vi "pythonHyperstack_CAllocated.vi"(1 "refresh_time":dbl=0.1, 2 "shape":i32[](array[numeric]), 3 "ptr":i64) -> (0 "ptr out":i64)   [LabVIEW 2017]
uses:
  globalUtilities.vi
  dll/wormUtilities/x64/Release/wormUtilities.dll
panel:
  out "return type":dbl
  out "Array 2":dbl[](array[numeric])
  out "Array":dbl[](array[numeric])
  out "result":bool
  out "shape 2":i32[](array[numeric])
  out "out":sgl[](array[numeric])
  out "Numeric":i32
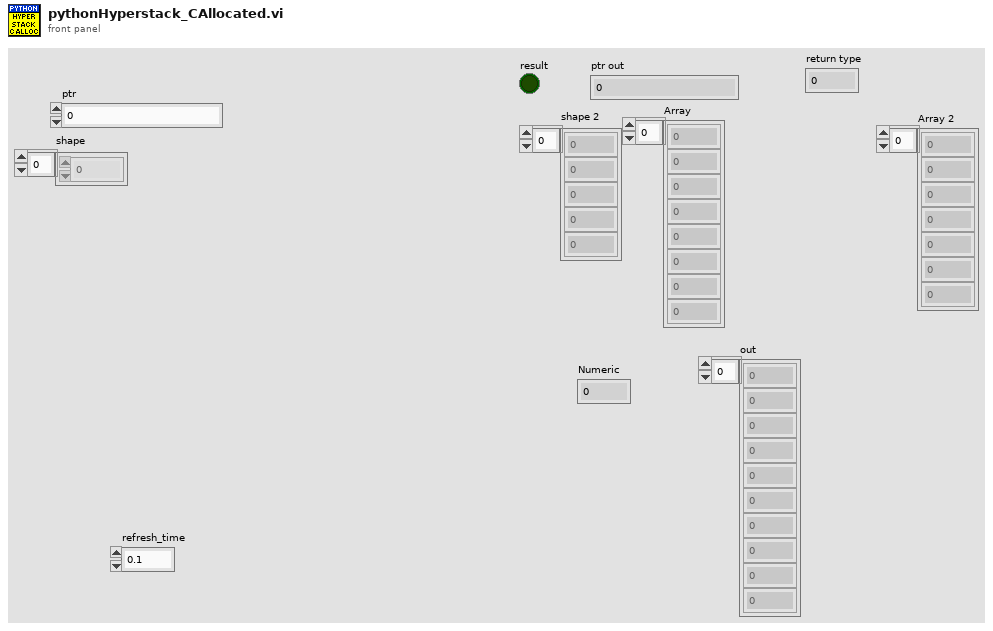
[diagram p1: front panel]
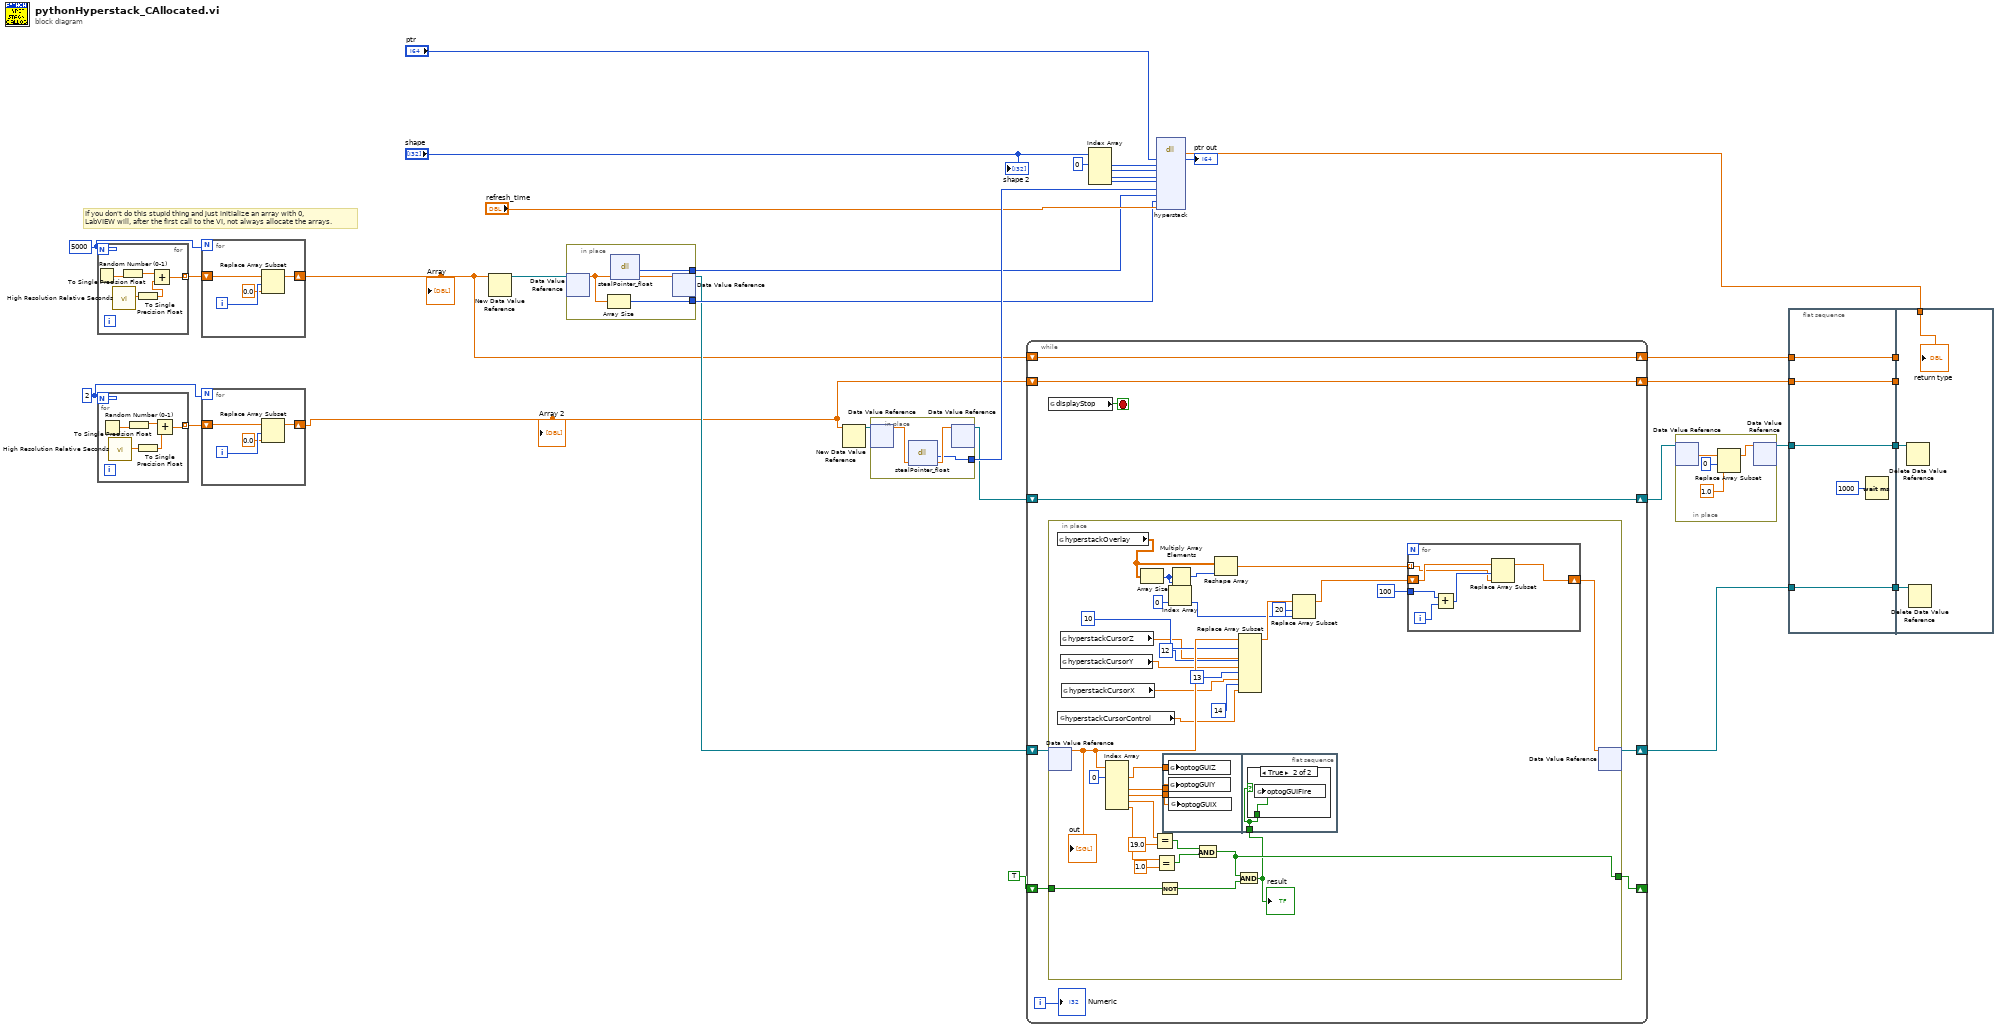
[diagram p0: block diagram]
diagram:
  w18 = 2
  w17 = 5000
  # "If you don't do this stupid thing and just initialize an array with 0, \nLabVIEW will, after the first call to the VI, not always allocate the arrays."
  n1 = for {
    N: w17 -> [_]
    tunnel: [w36] -> w22 mode=indexing
    n2 = Random Number (0-1)() -> (number: 0 to 1=w38:dbl)
    n3 = call <vilib>:"High Resolution Relative Seconds.vi"() -> ("relative seconds"=w35:dbl)
    n4 = To Single Precision Float(number=w38) -> (single precision float=w37:sgl)
    n5 = To Single Precision Float(number=w35) -> (single precision float=w34:sgl)
    n6 = Add(x=w37, y=w34) -> (x+y=w36:sgl)
  }
  n7 = for {
    N: w18 -> [_]
    tunnel: [w41] -> w20 mode=indexing
    n8 = Random Number (0-1)() -> (number: 0 to 1=w43:dbl)
    n9 = call <vilib>:"High Resolution Relative Seconds.vi"() -> ("relative seconds"=w40:dbl)
    n10 = To Single Precision Float(number=w43) -> (single precision float=w42:sgl)
    n11 = To Single Precision Float(number=w40) -> (single precision float=w39:sgl)
    n12 = Add(x=w42, y=w39) -> (x+y=w41:sgl)
  }
  n13 = for {
    N: w17 -> [_]
    shift-right: [w44] -> w21
    shift-left: w22 -> [w47]
    i -> [w46]
    n14 = Replace Array Subset(array=w47, new element=sgl 0.0 ("new element/subarray"), index=w46) -> (w44:sgl[])
  }
  "Array" <- w21
  n15 = for {
    N: w18 -> [_]
    shift-right: [w48] -> w19
    shift-left: w20 -> [w51]
    i -> [w50]
    n16 = Replace Array Subset(array=w51, new element=sgl 0.0 ("new element/subarray"), index=w50) -> (w48:sgl[])
  }
  "Array 2" <- w19
  n17 = New Data Value Reference(data value=w21) -> (data value reference=w26:refnum<data-value>)  [unwired: 1 in, 1 out]
  n18 = in-place {
    in-place-border: [w54] -> w28
    in-place-border: [w52] -> w27
    n19 = in-place-dvr #1(w26) -> (w53:sgl[])  [unwired: 1 out]
    n20 = Array Size(array=w53) -> (size(s)=w52:i32)
    n21 = dll-call lib="C:/Users/francesco/dev/pump-probe/dll/wormUtilities/x64/Release/wormUtilities.dll" fn="stealPointer_float"("A"=w53) -> ("return type"=w54:i64, "A"=w55:sgl[])  [unwired: 3 in, 2 out]
    n22 = in-place-dvr #1(w55) -> (w24:refnum<data-value>)  [unwired: 1 out]
  }
  n23 = New Data Value Reference(data value=w19) -> (data value reference=w32:refnum<data-value>)  [unwired: 1 in, 1 out]
  n24 = in-place {
    in-place-border: [w56] -> w33
    n25 = in-place-dvr #2(w32) -> (w57:sgl[])  [unwired: 1 out]
    n26 = dll-call lib="C:/Users/francesco/dev/pump-probe/dll/wormUtilities/x64/Release/wormUtilities.dll" fn="stealPointer_float"("A"=w57) -> ("return type"=w56:i64, "A"=w58:sgl[])  [unwired: 3 in, 2 out]
    n27 = in-place-dvr #2(w58) -> (w31:refnum<data-value>)  [unwired: 1 out]
  }
  n28 = while {
    shift-right: [w63] -> w25
    shift-left: w24 -> [w65]
    shift-right: [w66] -> w30
    shift-left: w31 -> [w66]
    shift-right: [w62] -> w15
    shift-left: w21 -> [w62]
    shift-right: [w61] -> w14
    shift-left: w19 -> [w61]
    shift-right: [w60] -> _
    shift-left: TRUE -> [w59]
    i -> [w64]
    stop <- w67 stop-if-true
    n29 = global read "globalUtilities.vi" "displayStop"() -> (w67:bool)
    n30 = in-place {
      in-place-border: [w89] -> w60
      in-place-border: w59 -> [w91]
      n31 = in-place-dvr #3(w65) -> (w87:sgl[])  [unwired: 1 out]
      "out" <- w87
      n32 = global read "globalUtilities.vi" "hyperstackOverlay"() -> (w77:dbl[][])
      n33 = global read "globalUtilities.vi" "hyperstackCursorControl"() -> (w79:sgl)
      n34 = global read "globalUtilities.vi" "hyperstackCursorY"() -> (w81:sgl)
      n35 = global read "globalUtilities.vi" "hyperstackCursorZ"() -> (w82:sgl)
      n36 = global read "globalUtilities.vi" "hyperstackCursorX"() -> (w80:sgl)
      n37 = Index Array(array=w87, index #1=0 ("index")) -> (element #1=w100:sgl, element #3=w99:sgl, element #4=w98:sgl, element #5=w97:sgl, element #6=w95:sgl)  [unwired: 5 in, 1 out]
      n38 = Array Size(array=w77) -> (size(s)=w73:i32[])
      n39 = Equal?(x=w97, y=sgl 19.0) -> (x = y?=w93:bool)
      n40 = Equal?(x=w95, y=sgl 1.0) -> (x = y?=w92:bool)
      n41 = Not(x=w91) -> (.not. x?=w90:bool)
      n42 = flat-sequence {
        tunnel: w100 -> [w110]
        tunnel: w99 -> [w109]
        tunnel: w98 -> [w108]
        tunnel: w88 -> [w111]
        frame #0 {
          n43 = global write "globalUtilities.vi" "optogGUIZ"(w110) -> ()
          n44 = global write "globalUtilities.vi" "optogGUIY"(w109) -> ()
          n45 = global write "globalUtilities.vi" "optogGUIX"(w108) -> ()
        }
        frame #1 {
          n46 = case shown="True" w111 {
            tunnel: w111 -> [_ w112]
            frame False {
            }
            frame True {
              n47 = global write "globalUtilities.vi" "optogGUIFire"(w112) -> ()
            }
          }
        }
      }
      n48 = Index Array(array=w73, index=0) -> (element=w70:i32)
      n49 = Multiply Array Elements(1:w73) -> (0:w78:i32)
      n50 = Compound Arithmetic op=AND(w93, w92) -> (w89:bool)
      n51 = Reshape Array(w77, w78) -> (w76:dbl[])
      n52 = And(x=w89, y=w90) -> (x .and. y?=w88:bool)
      "result" <- w88
      n53 = Replace Array Subset(array=w87, new element #1=w82, index #1=10 ("index"), new element #2=w81, index #2=12 ("index"), new element #3=w80, index #3=13 ("index"), new element #4=w79, index #4=14 ("index")) -> (w71:sgl[])
      n54 = Replace Array Subset(array=w71, new element=w70, index=20) -> (w68:sgl[])
      n55 = for {
        tunnel: w76 -> [w103] mode=indexing
        tunnel: 100 -> [w106]
        shift-right: [w102] -> w74
        shift-left: w68 -> [w105]
        i -> [w107]
        n56 = Add(x=w106, y=w107) -> (x+y=w104:i32)
        n57 = Replace Array Subset(array=w105, new element=w103, index=w104) -> (w102:sgl[])
      }
      n58 = in-place-dvr #3(w74) -> (w63:refnum<data-value>)  [unwired: 1 out]
    }
    "Numeric" <- w64
  }
  n59 = Index Array(array="shape", index #1=0 ("index")) -> (element #1=w10:i32, element #2=w9:i32, element #3=w8:i32, element #4=w7:i32)  [unwired: 3 in]
  n60 = dll-call lib="C:/Users/francesco/dev/pump-probe/dll/wormUtilities/x64/Release/wormUtilities.dll" fn="hyperstack"("A"="ptr", "shape0"=w10, "shape1"=w9, "shape2"=w8, "shape3"=w7, "stop"=w33, "out"=w28, "out_n"=w27, "refresh_time"="refresh_time") -> ("return type"=w16:dbl, "A"=→"ptr out":i64)  [unwired: 11 in, 2 out]
  n61 = in-place {
    n62 = in-place-dvr #4(w30) -> (w116:sgl[])  [unwired: 1 out]
    n63 = Replace Array Subset(array=w116, new element=sgl 1.0 ("new element/subarray"), index=0) -> (w113:sgl[])
    n64 = in-place-dvr #4(w113) -> (w23:refnum<data-value>)  [unwired: 1 out]
  }
  n65 = flat-sequence {
    tunnel: w14 -> [w118]
    tunnel: w15 -> [w119]
    tunnel: w23 -> [w120]
    tunnel: w25 -> [w121]
    tunnel: [w121] -> w4
    tunnel: [w120] -> w3
    tunnel: [w119] -> w2
    tunnel: [w118] -> w1
    tunnel: w16 -> [w122]
    tunnel: w4 -> [w124]
    tunnel: w3 -> [w123]
    tunnel: w2 -> [_]
    tunnel: w1 -> [_]
    frame #0 {
      n66 = Wait (ms)(milliseconds to wait=u32 1000) -> ()  [unwired: 1 out]
    }
    frame #1 {
      n67 = Delete Data Value Reference(data value reference=w123) -> ()  [unwired: 1 in, 2 out]
      n68 = Delete Data Value Reference(data value reference=w124) -> ()  [unwired: 1 in, 2 out]
      "return type" <- w122
    }
  }
  "shape 2" <- "shape"
